vi "Z Aux Open Eth.vi"(8 "error in (no error)":errorcluster caption="错误输入（无错误）", 10 "phandle":u32, 11 "ipaddr":string) -> (0 "error out":errorcluster caption="错误输出", 1 "function return":i32, 2 "phandle out":u32, 3 "ipaddr out":string)   [LabVIEW 2015, in "zauxdll.lvlib"]
doc: "int32 __stdcall ZAux_OpenEth(char *ipaddr, ZMC_HANDLE * phandle);"
uses:
  zauxdll.lvlib
  zauxdll.dll
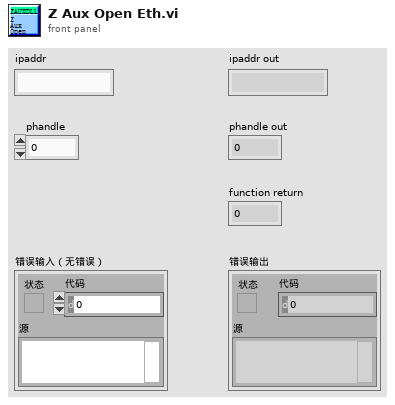
[diagram p1: front panel]
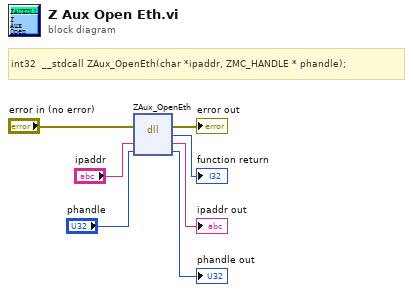
[diagram p0: block diagram]
diagram:
  # "int32  __stdcall ZAux_OpenEth(char *ipaddr, ZMC_HANDLE * phandle);"
  n1 = dll-call lib="D:/vicomm case/cub/0717/15/Main Folder/Radar - 2015 32bit_autoqueue_angle_0319/zauxdll-2014/zauxdll.*" fn="ZAux_OpenEth"(error in="error in (no error)", "ipaddr"="ipaddr", "phandle"="phandle") -> (error out=→"error out":errorcluster, "return type"=→"function return":i32, "ipaddr"=→"ipaddr out":string, "phandle"=→"phandle out":u32)  [unwired: 2 in, 1 out]
